vi "數值轉字串.vi"(1 "number":dbl) -> (0 "s? t:f":string)   [LabVIEW 2014]
uses:
  <vilib>/regexp/Match Regular Expression.xnode
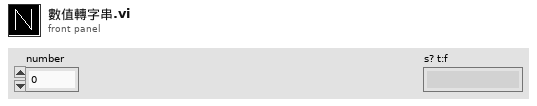
[diagram p1: front panel]
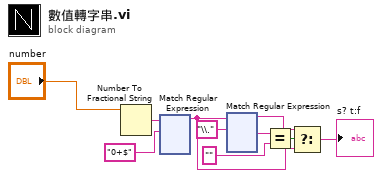
[diagram p0: block diagram]
diagram:
  n1 = Number To Fractional String(number="number") -> (F-format string=w9:string)  [unwired: 3 in]
  n2 = xnode "Match Regular Expression"("input string"=w9, "regular expression"="0+$") -> ("before match"=w3:string)  [unwired: 4 in, 4 out]
  n3 = xnode "Match Regular Expression"("input string"=w3, "regular expression"="\\.") -> ("before match"=w4:string, "after match"=w8:string)  [unwired: 4 in, 3 out]
  n4 = Equal?(x=w8, y="") -> (x = y?=w6:bool)
  n5 = Select(t=w4, s=w6, f=w3) -> (s? t:f=→"s? t:f":string)
